vi "APC_9056_MTRsignals.vi"(1 "PC_ControlSettings":T1={"Spark advance [CADBTDC]"=0.0, "Pref"=0.0, "O2ref"=0.0, "DI advance [CADBTDC]"=0.0, "DI duration [ms] "=0.0, "CO2ref"=0.0, "PFI duration [ms]"=0.0, "IMEP ref"=0.0, "Speed ref"=0.0, "IGN enable"=TRUE, "DI enable"=TRUE, "CL PFI\n lambda"=TRUE, "CL PFI\nIMEP"=FALSE, "Activate\ncylinder"=[FALSE, FALSE, FALSE, FALSE, FALSE, FALSE], "Force idling"=FALSE, "Force motoring"=FALSE, "ETP resync"=FALSE, "Requested mode"=0, "Clear Sync Errors"=FALSE, "toggle TDC"=FALSE, "l ref"=0.0, "PID control references"={"NG"=FALSE, "Ar"=FALSE, "O2"=FALSE, "Intake vent"=FALSE, "Cross vent"=FALSE, "Exhaust vent"=FALSE, "NG control mode"=0, "NG-FC-001-REF"=0.0, "WF-OA-002-REF"=0.0, "IMEP-REF"=0.0, "Nm-REF"=0.0, "Ar control mode"=0, "AR-PC-002-REF"=0.0, "WF-PT-004-REF"=0.0, "O2 control mode"=0, "O2-FC-001-REF"=0.0, "WF-OA-001-REF"=0.0, "Tcoolant control  mode"=0, "EC-FC-001-REF"=0.0, "EC-TT-001-REF"=0.0, "Texh control mode"=0, "SW-FC-004-REF"=0.0, "SW-FT-002-REF"=0.0, "WF-TT-004-REF"=0.0, "Toil control mode"=0, "SW-FC-009-REF"=0.0, "SW-FT-004-REF"=0.0, "EO-TT-001-REF"=0.0, "AIC201_CO2_ConcTarget"=0.0, "O2_FF_NG"=FALSE, "Dyno control mode"=0, "Membrane control mode"=0, "AR-FT-001-REF"=0.0, "MTR modbus floats"=[0.0, 0.0, 0.0, 0.0, 0.0, 0.0, 0.0, 0.0, 0.0, 0.0, 0.0, 0.0, 0.0, 0.0, 0.0, 0.0, 0.0, 0.0, 0.0], "MTR modbus u16"=[0, 0, 0, 0, 0, 0, 0], "MTR HB"=FALSE, "PC_HB"=FALSE, "EMERGENCY STOP"=FALSE}, "CA50setpoint [CADATDC]"=0.0, "CA50 control"=TRUE, "Knock control"=TRUE, "CLEAR EMERGENCY STOP"=FALSE, "EMERGENCY STOP"=FALSE}) -> (0 "MTR signals array":dbl[](array[numeric]))   [LabVIEW 2020]
uses:
  controls/APC_ControlSettings.ctl
  controls/APC_PIDcontrolSettings.ctl
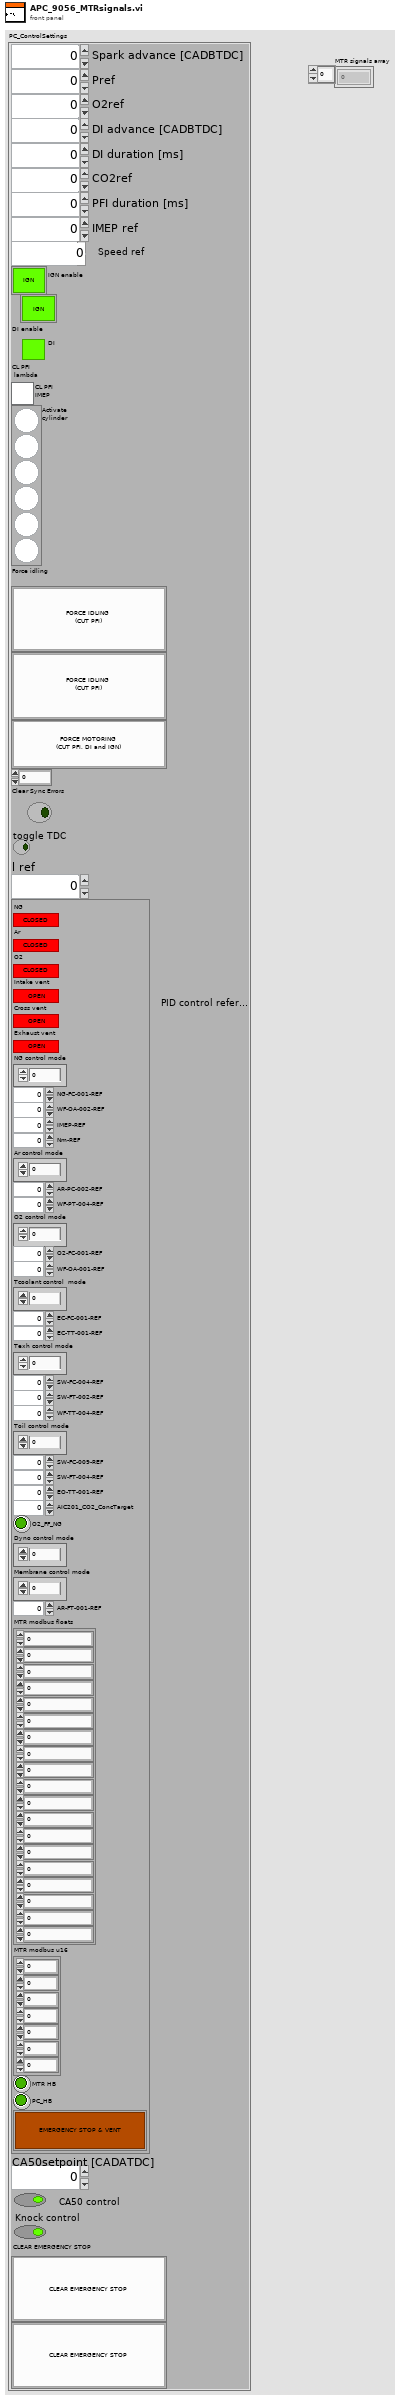
[diagram p1: front panel]
types:
  T1 = typedef "APC_ControlSettings.ctl" = cluster{"Spark advance [CADBTDC]":dbl, "Pref":dbl, "O2ref":dbl, "DI advance [CADBTDC]":dbl, "DI duration [ms] ":dbl, "CO2ref":dbl, "PFI duration [ms]":dbl, "IMEP ref":dbl, "Speed ref":dbl, "IGN enable":bool, "DI enable":bool, "CL PFI\n lambda":bool, "CL PFI\nIMEP":bool, "Activate\ncylinder":bool[], "Force idling":bool, "Force motoring":bool, "ETP resync":bool, "Requested mode":i8, "Clear Sync Errors":bool, "toggle TDC":bool, "l ref":dbl, "PID control references":T2, "CA50setpoint [CADATDC]":dbl, "CA50 control":bool, "Knock control":bool, "CLEAR EMERGENCY STOP":bool, "EMERGENCY STOP":bool}
  T2 = typedef "APC_PIDcontrolSettings.ctl" = cluster{"NG":bool, "Ar":bool, "O2":bool, "Intake vent":bool, "Cross vent":bool, "Exhaust vent":bool, "NG control mode":u8, "NG-FC-001-REF":dbl, "WF-OA-002-REF":dbl, "IMEP-REF":dbl, "Nm-REF":dbl, "Ar control mode":u8, "AR-PC-002-REF":dbl, "WF-PT-004-REF":dbl, "O2 control mode":u8, "O2-FC-001-REF":dbl, "WF-OA-001-REF":dbl, "Tcoolant control  mode":u8, "EC-FC-001-REF":dbl, "EC-TT-001-REF":dbl, "Texh control mode":u8, "SW-FC-004-REF":dbl, "SW-FT-002-REF":dbl, "WF-TT-004-REF":dbl, "Toil control mode":u8, "SW-FC-009-REF":dbl, "SW-FT-004-REF":dbl, "EO-TT-001-REF":dbl, "AIC201_CO2_ConcTarget":dbl, "O2_FF_NG":bool, "Dyno control mode":u8, "Membrane control mode":u8, "AR-FT-001-REF":dbl, "MTR modbus floats":sgl[], "MTR modbus u16":u16[], "MTR HB":bool, "PC_HB":bool, "EMERGENCY STOP":bool}
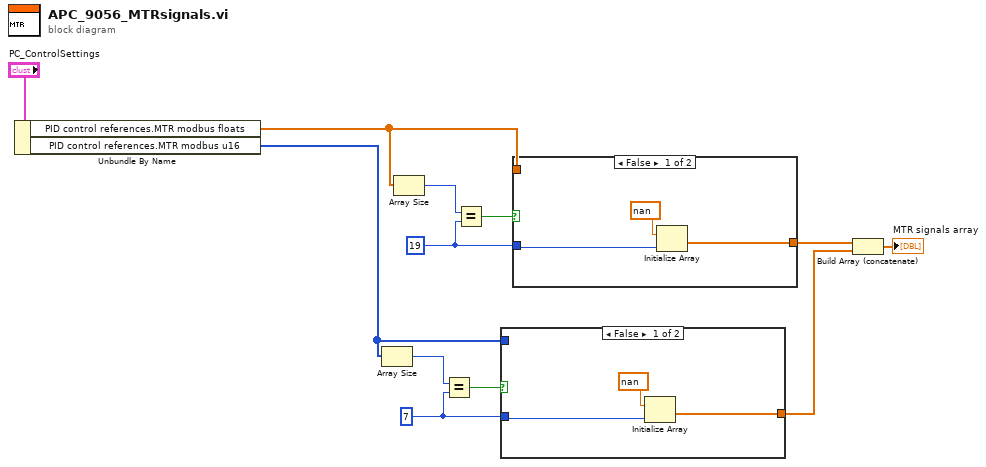
[diagram p0: block diagram]
diagram:
  w5 = 7 ("y")
  w8 = 19 ("y")
  n1 = Unbundle By Name("PC_ControlSettings") -> ("PID control references.MTR modbus floats"=w9:sgl[], "PID control references.MTR modbus u16"=w4:u16[])
  n2 = Array Size(array=w4) -> (size(s)=w7:i32)
  n3 = Array Size(array=w9) -> (size(s)=w12:i32)
  n4 = Equal?(x=w7, y=w5) -> (x = y?=w6:bool)
  n5 = Equal?(x=w12, y=w8) -> (x = y?=w11:bool)
  n6 = case shown="False" w6 {
    tunnel: w4 -> [_ w16]
    tunnel: w5 -> [w15 _]
    tunnel: [w13 w16] -> w2
    frame False {
      n7 = Initialize Array(nan ("element"), w15) -> (w13:dbl[])
    }
    frame True {
    }
  }
  n8 = case shown="False" w11 {
    tunnel: w9 -> [_ w20]
    tunnel: w8 -> [w19 _]
    tunnel: [w17 w20] -> w3
    frame False {
      n9 = Initialize Array(nan ("element"), w19) -> (w17:dbl[])
    }
    frame True {
    }
  }
  n10 = Build Array (concatenate)(w3, w2) -> (→"MTR signals array":dbl[])
